vi "Dataset Source 2 Types.vi"(6 "Hold":T2, 10 "Dataset Source":T3) -> (2 "Types":T1[](array[typedef]))   [LabVIEW 2009]
uses:
  Dataset Source.ctl
  Dataset Type.ctl
  Apps/Yes No Button.ctl
panel:
  in  "Hold Types":T1[](array[typedef])=[enum."Displacement", enum."Force"]
  in  "External Sensor Types":T1[](array[typedef])=[enum."LVDT"]
  in  "Combined Types":T1[](array[typedef])=[enum."Displacement Command", enum."Displacement", enum."Force"]
  in  "LBCB  Types":T1[](array[typedef])=[enum."Actuator Command", enum."LVDT", enum."Load Cell", enum."Servo Error", enum."Displacement Command", enum."Displacement", enum."Force"]
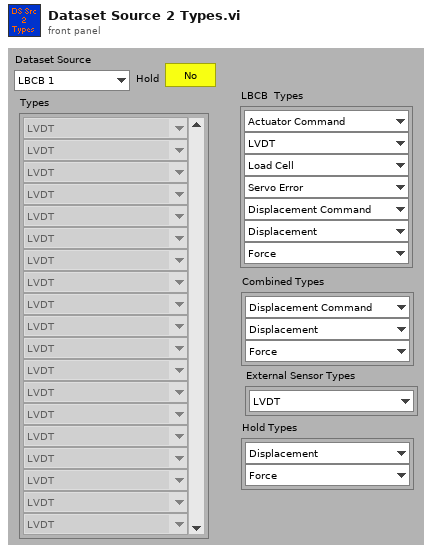
[diagram p1: front panel]
types:
  T1 = typedef "Dataset Type.ctl" = enum16{"LVDT", "Load Cell", "Actuator Command", "Servo Error", "Displacement Command", "Displacement", "Force"}
  T2 = typedef "Yes No Button.ctl" = bool
  T3 = typedef "Dataset Source.ctl" = enum16{"LBCB 1", "LBCB 2", "Combined", "External Sensors"}
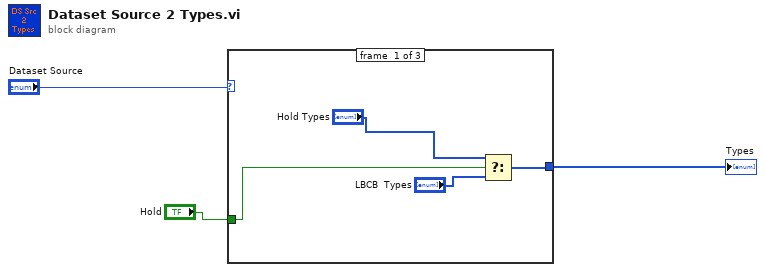
[diagram p0: block diagram]
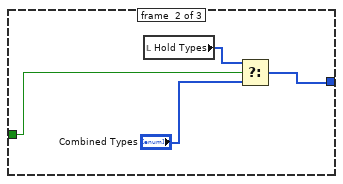
[diagram p2: hidden frame]
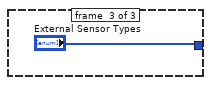
[diagram p3: hidden frame]
diagram:
  n1 = case shown="\"Combined\"" "Dataset Source" {
    tunnel: [w5 w10 "External Sensor Types"] -> w2
    tunnel: "Hold" -> [w6 w9 _]
    frame #0 {
      n2 = Select(t="Hold Types", s=w6, f="LBCB  Types") -> (s? t:f=w5:T1[])
    }
    frame #1 {
      n3 = local read "Hold Types"() -> (w8:T1[])
      n4 = Select(t=w8, s=w9, f="Combined Types") -> (s? t:f=w10:T1[])
    }
    frame #2 {
    }
  }
  "Types" <- w2
